vi "MarkTested.vi"(7 "Enum":enum16{"MarkTested", "MarkNotTested"}(ring), 8 "error in (no error)":errorcluster, 11 "LotData in":refnum<class "LotData.lvclass">) -> (0 "error out":errorcluster, 2 "Message":string, 3 "LotData out":refnum<class "LotData.lvclass">)   [LabVIEW 2012, in "LotData.lvclass"]
uses:
  LotData.lvclass
  <vilib>/addons/database/NI_Database_API.lvlib
  <vilib>/addons/database/Connection.llb/DB Tools Open Connec (Path).vi
  <vilib>/addons/database/Command.llb/Cmd Set Parameter Value (C).vi
  <vilib>/addons/database/Command.llb/Cmd Execute.vi
  <vilib>/addons/database/Recordset.llb/Rec Destroy - Command.vi
  <vilib>/addons/database/Command.llb/Cmd Delete.vi
  <vilib>/addons/database/Auxilliary.llb/DB Tools Parameter Dir.ctl
  <vilib>/addons/database/Auxilliary.llb/DB Tools DataTypes.ctl
  <vilib>/addons/database/Auxilliary.llb/DB Tools Parameter Info.ctl
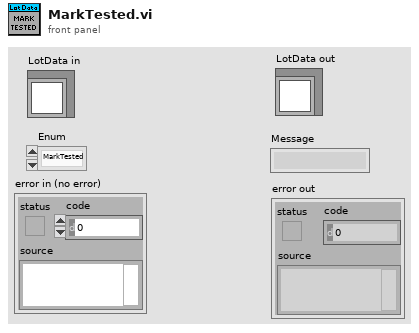
[diagram p1: front panel]
types:
  T1 = typedef "NI_Database_API.lvlib/DB Tools Parameter Info.ctl" = cluster{"parameter name":string, "type":T2, "direction":T3, "value":variant}
  T2 = typedef "NI_Database_API.lvlib/DB Tools DataTypes.ctl" = enum16{"String", "Long (I32)", "Single (SGL)", "Double (DBL)", "Date/Time", "Binary"}
  T3 = typedef "NI_Database_API.lvlib/DB Tools Parameter Dir.ctl" = enum32{"Input", "Output", "Input/Output", "Return Value"}
  T4 = typedef "MeasurementType.ctl" = enum16{"Initial", "Final"}
  T5 = typedef "NI_Database_API.lvlib/Conn ObjectReference.ctl" = refnum<k1>
  T6 = typedef "NI_Database_API.lvlib/Cmd ObjectReference.ctl" = refnum<k1>
  T7 = typedef "NI_Database_API.lvlib/Cmd-Rec Object Reference.ctl" = refnum<k1>
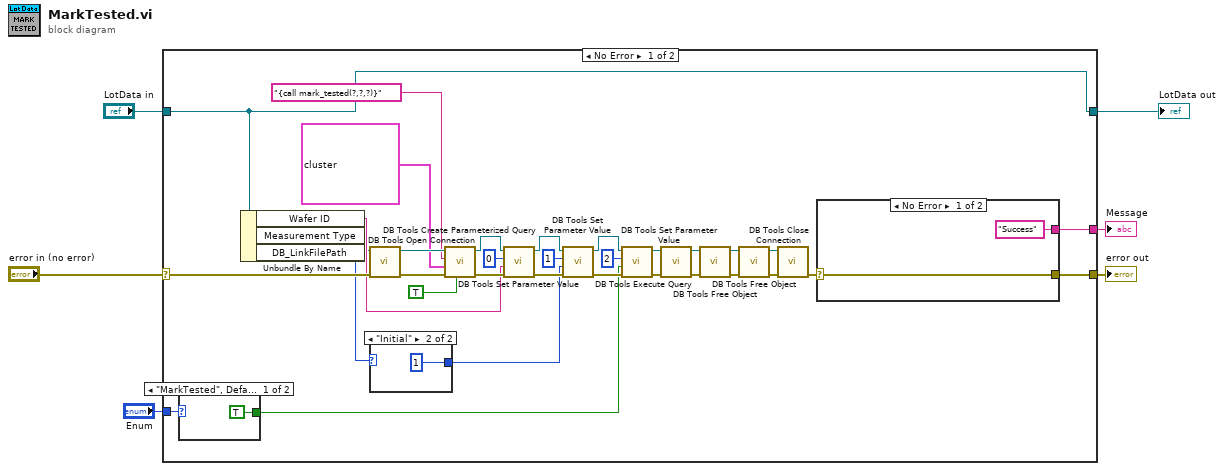
[diagram p0: block diagram]
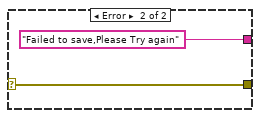
[diagram p2: hidden frame]
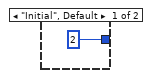
[diagram p3: hidden frame]
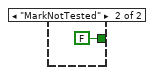
[diagram p4: hidden frame]
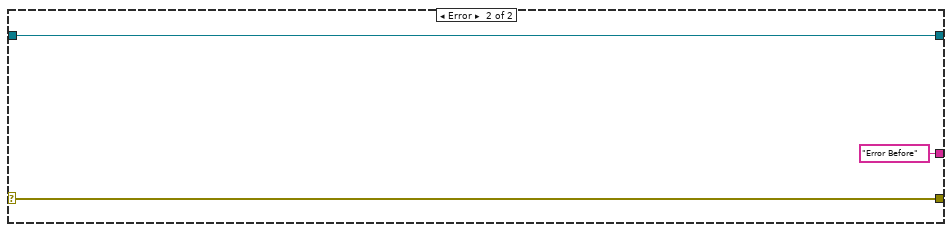
[diagram p5: hidden frame]
diagram:
  n1 = case shown="No Error" "error in (no error)" {
    selector: "error in (no error)" -> [w15 w50]
    tunnel: [w8 w50] -> w5
    tunnel: [w38 w48] -> w3
    tunnel: "LotData in" -> [w38 w48]
    tunnel: "Enum" -> [w39 _]
    tunnel: [w9 "Error Before"] -> w1
    frame No Error {
      n2 = case shown="\"MarkTested\", Default" w39 {
        tunnel: [TRUE ("isTested") FALSE ("isTested")] -> w13
        frame "MarkTested", Default {
        }
        frame "MarkNotTested" {
        }
      }
      n3 = Unbundle By Name(w38) -> ("Wafer ID"=w14:string, "Measurement Type"=w12:T4, "DB_LinkFilePath"=w7:path)
      n4 = call-poly <vilib>:"DB Tools Open Connection.vi"("error in (no error)"=w15, "connection information"=w7) -> ("error out"=w35:errorcluster, "connection reference"=w36:T5)  [unwired: 6 in]
      n5 = case shown="\"Initial\"" w12 {
        tunnel: [2 1] -> w11
        frame "Initial", Default {
        }
        frame "Initial" {
        }
      }
      n6 = call <vilib>:"DB Tools Create Parameterized Query.vi"("stored procedure? (F)"=TRUE, "error in (no error)"=w35, "parameters"=T1[] [{"parameter name"="wafer", "type"=enum."String", "direction"=enum."Input", "value"=variant}, {"parameter name"="test", "type"=enum."Single (SGL)", "direction"=enum."Input", "value"=variant}, {"parameter name"="isTested", "type"=enum."Binary", "direction"=enum."Input", "value"=variant}], "SQL query"="{call mark_tested(?,?,?)}", "connection reference"=w36) -> ("error out"=w32:errorcluster, "command reference"=w31:T6)  [unwired: 2 in, 1 out]
      n7 = call-poly <vilib>:"DB Tools Set Parameter Value.vi"("error in (no error)"=w32, "value"=w14, "parameter index"=0, "command reference"=w31) -> ("error out"=w24:errorcluster, "command reference out"=w23:T6)  [unwired: 4 in]
      n8 = call-poly <vilib>:"DB Tools Set Parameter Value.vi"("error in (no error)"=w24, "value"=w11, "parameter index"=1, "command reference"=w23) -> ("error out"=w21:errorcluster, "command reference out"=w22:T6)  [unwired: 4 in]
      n9 = call-poly <vilib>:"DB Tools Set Parameter Value.vi"("error in (no error)"=w21, "value"=w13, "parameter index"=2, "command reference"=w22) -> ("error out"=w16:errorcluster, "command reference out"=w17:T6)  [unwired: 4 in]
      n10 = call-poly <vilib>:"DB Tools Execute Query.vi"("error in (no error)"=w16, "command reference"=w17) -> ("error out"=w28:errorcluster, "command-recordset reference"=w29:T7)  [unwired: 6 in]
      n11 = call-poly <vilib>:"DB Tools Free Object.vi"("error in (no error)"=w28, "command-recordset reference"=w29) -> ("error out"=w30:errorcluster, "command reference"=w25:T6)  [unwired: 8 in]
      n12 = call-poly <vilib>:"DB Tools Free Object.vi"("error in (no error)"=w30, "command reference"=w25) -> ("error out"=w26:errorcluster, "connection reference"=w27:T5)  [unwired: 8 in]
      n13 = call <vilib>:"DB Tools Close Connection.vi"("error in (no error)"=w26, "connection reference"=w27) -> ("error out"=w10:errorcluster)  [unwired: 5 in]
      n14 = case shown="No Error" w10 {
        selector: w10 -> [w40 w43]
        tunnel: ["Success" "Failed to save,Please Try again"] -> w9
        tunnel: [w40 w43] -> w8
        frame No Error {
        }
        frame Error {
        }
      }
    }
    frame Error {
    }
  }
  "error out" <- w5
  "LotData out" <- w3
  "Message" <- w1
